vi "Get Children Recursively.vi"(8 "error in (no error)":errorcluster, 10 "All Data":refnum<class "Data Item.lvclass">[](array[class]), 11 "Data Item in":refnum<class "Data Item.lvclass">) -> (0 "error out":errorcluster, 1 "Children Indices":i32[](array[numeric]), 2 "Children":refnum<class "Data Item.lvclass">[](array[class]), 3 "Data Item out":refnum<class "Data Item.lvclass">)   [LabVIEW 2026, in "VILab.lvlib" / "Data Item.lvclass"]
uses:
  Data Item.lvclass
  Data Item.lvclass/Data Item.ctl
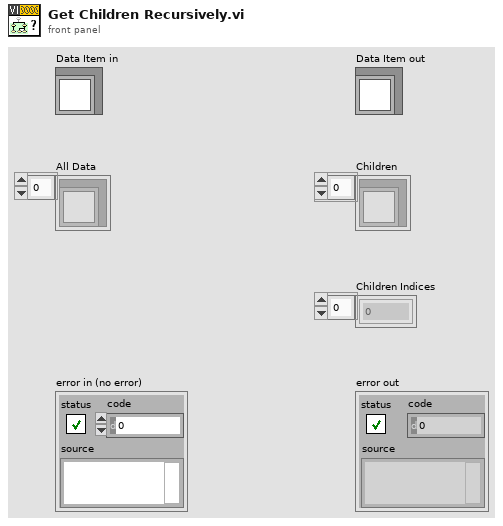
[diagram p1: front panel]
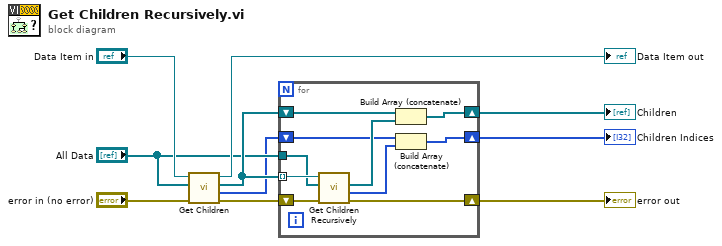
[diagram p0: block diagram]
diagram:
  n1 = call-dynamic "Get Children.vi"("error in (no error)"="error in (no error)", "All Data"="All Data", "Data Item in"="Data Item in") -> ("error out"=w5:errorcluster, "Children Indices"=w2:i32[], "Children"=w4:refnum<class "Data Item.lvclass">[], "Data Item out"=→"Data Item out":refnum<class "Data Item.lvclass">)  [unwired: 5 in]
  n2 = for {
    tunnel: w4 -> [w15] mode=indexing
    shift-right: [w19] -> w9
    shift-left: w5 -> [w20]
    shift-right: [w16] -> w6
    shift-left: w4 -> [w18]
    tunnel: "All Data" -> [w14]
    shift-right: [w11] -> w1
    shift-left: w2 -> [w13]
    n3 = call "Get Children Recursively.vi"("error in (no error)"=w20, "All Data"=w14, "Data Item in"=w15) -> ("error out"=w19:errorcluster, "Children Indices"=w12:i32[], "Children"=w17:refnum<class "Data Item.lvclass">[])  [unwired: 5 in, 1 out]
    n4 = Build Array (concatenate)(w18, w17) -> (w16:refnum<class "Data Item.lvclass">[])
    n5 = Build Array (concatenate)(w13, w12) -> (w11:i32[])
  }
  "error out" <- w9
  "Children" <- w6
  "Children Indices" <- w1
